vi "Decode Data.vi"(8 "Error In":errorcluster, 10 "Buffer":u8[](array[numeric]), 11 "Read":i32) -> (0 "Error Out":errorcluster, 3 "ToString":string)   [LabVIEW 2014, in "SSL Lib.lvlib"]
uses:
  <userlib>/SSL Library/SSL Lib.lvlib
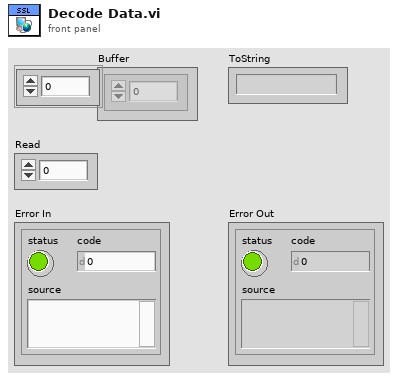
[diagram p1: front panel]
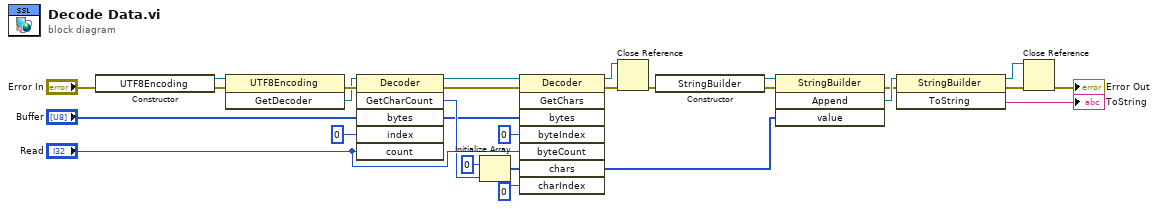
[diagram p0: block diagram]
diagram:
  n1 = constructor class="UTF8Encoding"(error in="Error In") -> (reference out=w4:refnum<k24>, error out=w3:errorcluster)  [unwired: 2 in, 1 out]
  n2 = invoke class="UTF8Encoding" method="GetDecoder"(reference=w4, error in=w3) -> (error out=w2:errorcluster, "GetDecoder"=w1:refnum<k24>)  [unwired: 1 in, 1 out]
  n3 = invoke class="Decoder" method="GetCharCount"(reference=w1, error in=w2, "bytes"="Buffer", "index"=0, "count"="Read") -> (reference out=w6:refnum<k24>, error out=w7:errorcluster, "GetCharCount"=w14:i32, "bytes"=w8:u8[])  [unwired: 1 in, 2 out]
  n4 = Initialize Array(u16 0 ("element"), w14) -> (w16:u16[])
  n5 = invoke class="Decoder" method="GetChars"(reference=w6, error in=w7, "bytes"=w8, "byteIndex"=0, "byteCount"="Read", "chars"=w16, "charIndex"=0 ("byteIndex")) -> (reference out=w27:refnum<k24>, error out=w24:errorcluster, "chars"=w18:u16[])  [unwired: 1 in, 5 out]
  n6 = Close Reference(reference=w27, error in (no error)=w24) -> (error out=w25:errorcluster)
  n7 = constructor class="StringBuilder"(error in=w25) -> (reference out=w12:refnum<k24>, error out=w9:errorcluster)  [unwired: 2 in, 1 out]
  n8 = invoke class="StringBuilder" method="Append"(reference=w12, error in=w9, "value"=w18) -> (error out=w10:errorcluster, "Append"=w11:refnum<k24>)  [unwired: 1 in, 2 out]
  n9 = invoke class="StringBuilder" method="ToString"(reference=w11, error in=w10) -> (reference out=w23:refnum<k24>, error out=w21:errorcluster, "ToString"=→"ToString":string)  [unwired: 1 in]
  n10 = Close Reference(reference=w23, error in (no error)=w21) -> (error out=→"Error Out":errorcluster)
